vi "Point&Path@Select(X=A_B_C)__Parameter.vi"(1 "ParamterIn":string) -> (0 "ParamterOut":string)   [LabVIEW 2020]
panel:
  in  "C":string(combo)
  in  "B":string(combo)
  in  "Logic":string(combo)
  in  "X":string(combo)
  in  "Confirm":bool
  # "Point&Path@Select(X=A?B:C)"
  # "True"
  # "="
  # "False"
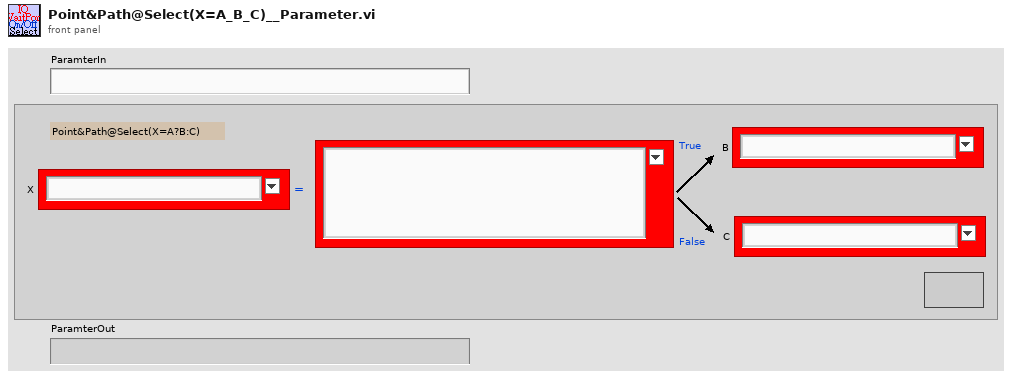
[diagram p1: front panel]
types:
  T1 = enum16{"Get", "UpdatePointS", "Init", "UpdateIndex", "GetCurrent&Index+1", "GetWithIndex", "ChkLast", "GetCurrent"}
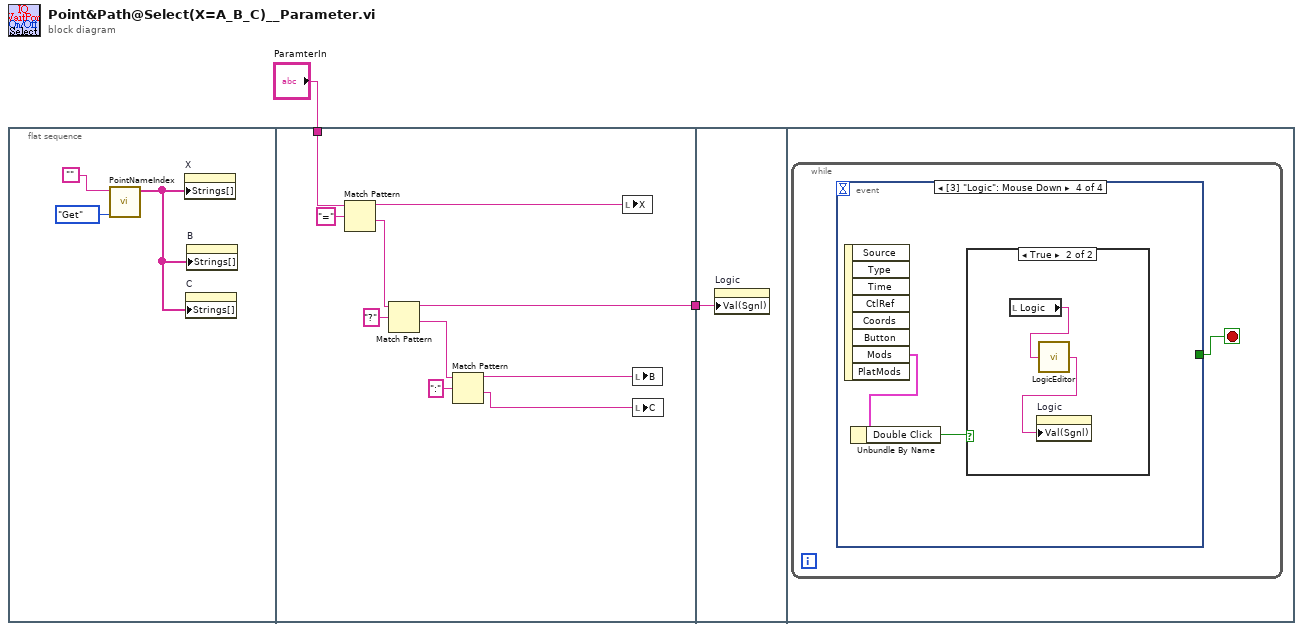
[diagram p0: block diagram]
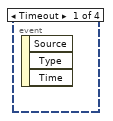
[diagram p2: hidden frame]
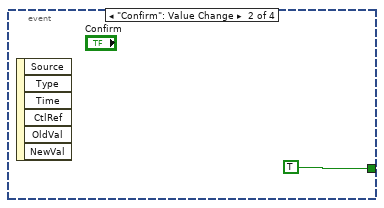
[diagram p3: hidden frame]
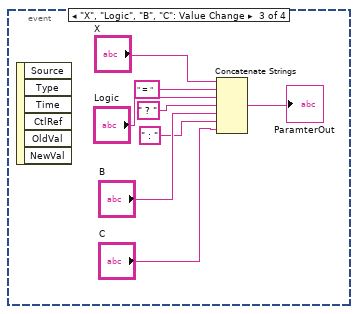
[diagram p4: hidden frame]
diagram:
  n1 = flat-sequence {
    tunnel: "ParamterIn" -> [w15]
    tunnel: [w10] -> w1
    tunnel: w1 -> [w16]
    frame #0 {
      n2 = call "PointNameIndex.vi"("OP"=T1."Get", "PointName"="") -> ("PointNameList"=w3:string[])  [unwired: 4 in, 5 out]
      n3 = property on="X" class="CmbBox"("Strings[]"=w3) -> ()  [unwired: 2 in, 2 out]
      n4 = property on="C" class="CmbBox"("Strings[]"=w3) -> ()  [unwired: 2 in, 2 out]
      n5 = property on="B" class="CmbBox"("Strings[]"=w3) -> ()  [unwired: 2 in, 2 out]
    }
    frame #1 {
      n6 = Match Pattern(string=w15, regular expression="=") -> (before substring=w13:string, after substring=w12:string)  [unwired: 1 in, 2 out]
      n7 = Match Pattern(string=w12, regular expression="?") -> (before substring=w10:string, after substring=w9:string)  [unwired: 1 in, 2 out]
      n8 = Match Pattern(string=w9, regular expression=":") -> (before substring=w7:string, after substring=w6:string)  [unwired: 1 in, 2 out]
      n9 = local write "X"(w13) -> ()
      n10 = local write "B"(w7) -> ()
      n11 = local write "C"(w6) -> ()
    }
    frame #2 {
      n12 = property on="Logic" class="CmbBox"("Val(Sgnl)"=w16) -> ()  [unwired: 2 in, 2 out]
    }
    frame #3 {
      n13 = while {
        stop <- w17 stop-if-true
        n14 = event shown="[3] \"Logic\": Mouse Down" {
          selector: _ -> [_ _ _ _]
          dyn-events: _ -> [_ _ _ _]
          timeout: _ -> [_ _ _ _]
          tunnel: [_ TRUE _ _] -> w17
          event Timeout {
            n15 = event-data() -> ()  [unwired: 1 in, 3 out]
          }
          event "Confirm": Value Change {
            n16 = event-data() -> ()  [unwired: 1 in, 6 out]
          }
          event "X", "Logic", "B", "C": Value Change {
            n17 = event-data() -> ()  [unwired: 1 in, 6 out]
            n18 = Concatenate Strings("X", " = " ("string"), "Logic", " ? " ("string"), "B", " : " ("string"), "C") -> (→"ParamterOut":string)
          }
          event "Logic": Mouse Down {
            n19 = event-data() -> ("Mods"=w28:cluster{"Double Click":bool, "Menu Key":bool})  [unwired: 1 in, 7 out]
            n20 = Unbundle By Name(w28) -> ("Double Click"=w27:bool)
            n21 = case shown="True" w27 {
              frame False {
              }
              frame True {
                n22 = local read "Logic"() -> (w30:string)
                n23 = call "LogicEditor.vi"("Logic Express"=w30) -> ("LogicExpressOut"=w29:string)
                n24 = property on="Logic" class="CmbBox"("Val(Sgnl)"=w29) -> ()  [unwired: 2 in, 2 out]
              }
            }
          }
        }
      }
    }
  }
